vi "AddModule.vi"(4 "python module name":string, 5 "python module":string, 6 "error in":errorcluster, 9 "PythonConverter_BD in":refnum<class "PyConvBD.lvclass">) -> (0 "error out":errorcluster, 3 "PythonConverter_BD out":refnum<class "PyConvBD.lvclass">)   [LabVIEW 2014, in "Raspberry Pi Compatible Compiler for LabVIEW.lvlib" / "PyConvBD.lvclass"]
uses:
  PyConvBD.lvclass
  PyConvBD.lvclass/PyConvBD.ctl
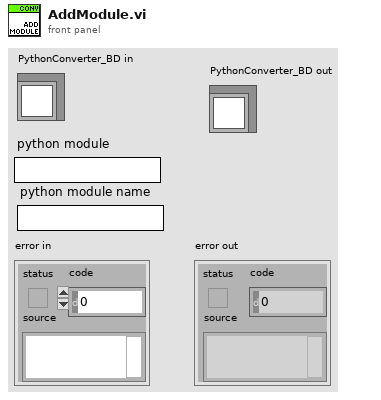
[diagram p1: front panel]
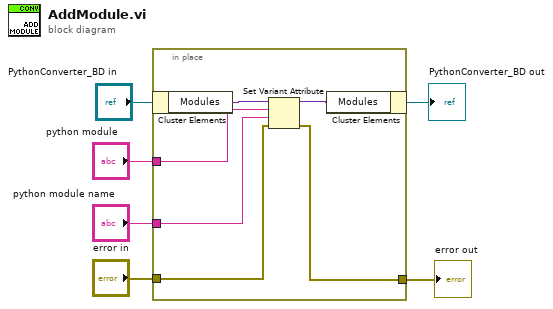
[diagram p0: block diagram]
diagram:
  n1 = in-place {
    in-place-border: "error in" -> [w11]
    in-place-border: [w10] -> w2
    in-place-border: "python module" -> [w9]
    in-place-border: "python module name" -> [w8]
    n2 = in-place-cluster #1("PythonConverter_BD in") -> ("Modules"=w7:variant)
    n3 = Set Variant Attribute(Variant=w7, name=w9, value=w8, error in=w11) -> (Variant out=w12:variant, error out=w10:errorcluster)  [unwired: 1 out]
    n4 = in-place-cluster #1("Modules"=w12) -> (→"PythonConverter_BD out":refnum<class "PyConvBD.lvclass">)
  }
  "error out" <- w2
